vi "test ramp.vi"() -> ()   [LabVIEW 2015]
uses:
  model type.ctl
  coag.ctl
panel:
  out "Waveform Chart":dbl(graph)
  in  "milliseconds to wait":u32
  out "Coag dose":dbl
  in  "Coagulant":T1={"flocculator volume (L)"=100.0, "clarifier volume (L)"=0.0, "dose updates per HRT"=0, "target clarified turbidity (NTU)"=0.3, "Coagulant mode"=enum."manual", "Coag dose [mg/L]"=0.0, "pump mL/rev"=0.0, "clarifier flow [L/s]"=0.5, "min Coag dose [mg/L]"=0.0, "max Coag dose [mg/L]"=0.0, "Steps"=3, "HRT response delay"=1, "Ku*"=1.0} {"HRT response delay" min=1 max=10 step=1; "Steps" min=3 step=1; "clarifier flow [L/s]" min=0.0001 max=1.0 step=0.0001; "target clarified turbidity (NTU)" min=0.1 max=5.0 step=0.01; "dose updates per HRT" min=1 max=100 step=1}
  in  "stop":bool
  # "min"
  # "max"
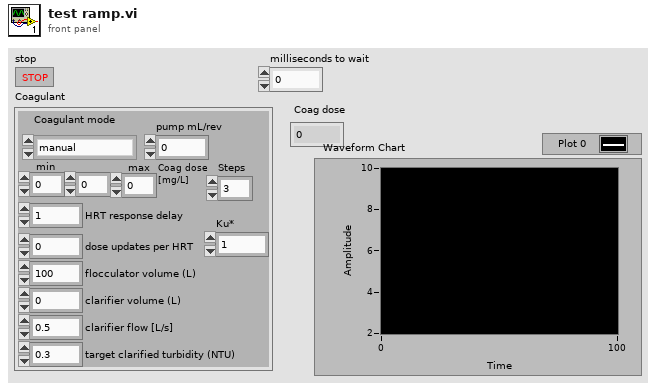
[diagram p1: front panel]
types:
  T1 = typedef "coag.ctl" = cluster{"flocculator volume (L)":dbl, "clarifier volume (L)":dbl, "dose updates per HRT":u16, "target clarified turbidity (NTU)":dbl, "Coagulant mode":T2, "Coag dose [mg/L]":dbl, "pump mL/rev":dbl, "clarifier flow [L/s]":dbl, "min Coag dose [mg/L]":dbl, "max Coag dose [mg/L]":dbl, "Steps":u16, "HRT response delay":u32, "Ku*":dbl}
  T2 = typedef "model type.ctl" = enum16{"manual", "ramp", "simple corrector", "linear regression"}
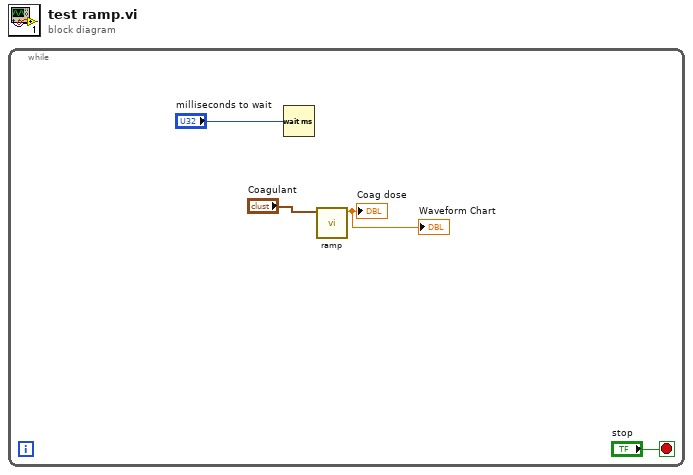
[diagram p0: block diagram]
diagram:
  n1 = while {
    stop <- "stop" stop-if-true
    n2 = Wait (ms)(milliseconds to wait="milliseconds to wait") -> ()  [unwired: 1 out]
    n3 = call "ramp.vi"("Coagulant"="Coagulant") -> ("Coag dose"=→"Coag dose" →"Waveform Chart":dbl)  [unwired: 10 in]
  }
